vi "MinDisplac(StartP)1.vi"(4 "error IN":errorcluster, 7 "[IN] (X,Y,dX,dY) NN":dbl[][](array[numeric])) -> (0 "error OUT":errorcluster, 3 "[OUT] (X,Y,dX,dY) NN":dbl[][](array[numeric]))   [LabVIEW 2013]
doc: "If origins of displacement have the same coordinates, this subVI saves only minimal"
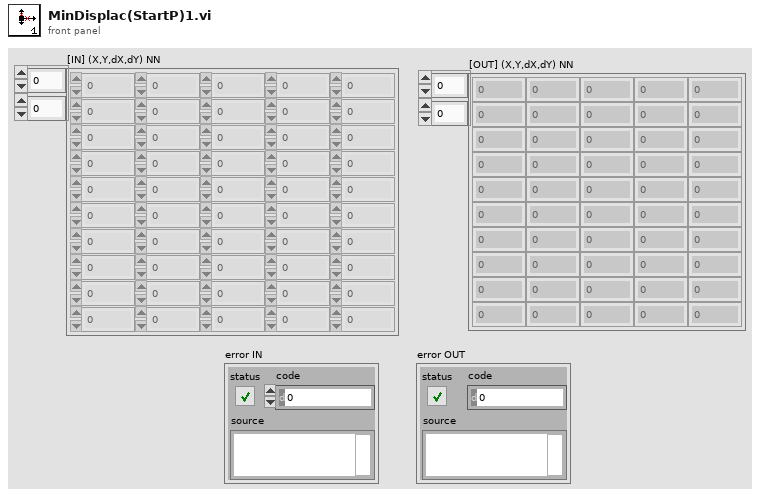
[diagram p1: front panel]
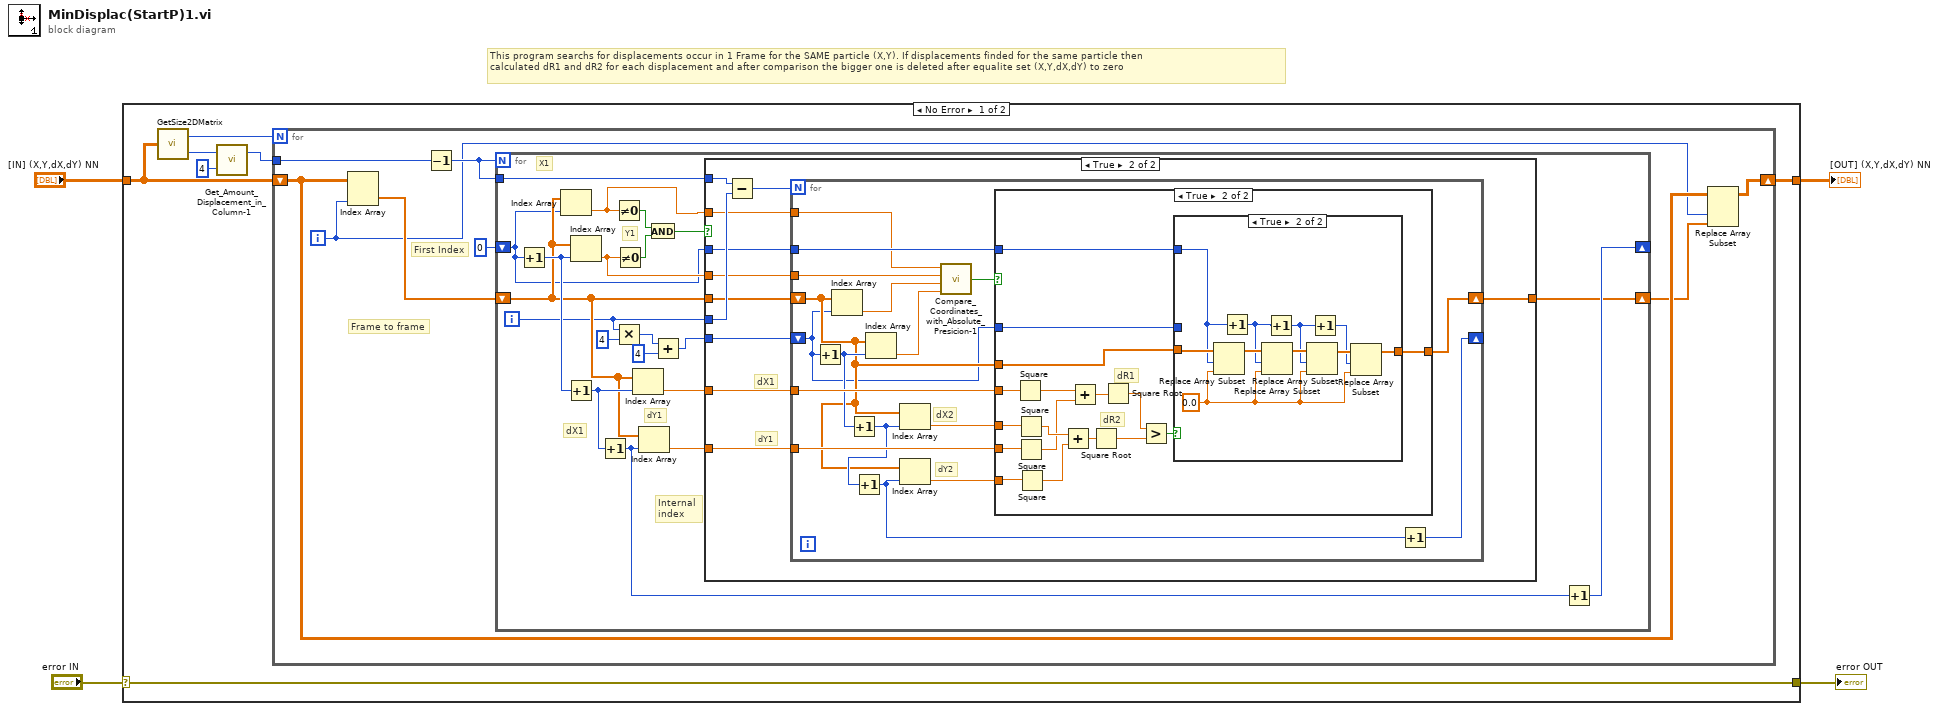
[diagram p0: block diagram]
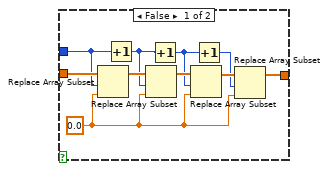
[diagram p4: hidden frame]
diagram:
  # "This program searchs for displacements occur in 1 Frame for the SAME particle (X,Y). If displacements finded for the same particle then \ncalculated dR1 and dR2 for each displacement and after comparison the bigger one is deleted after equalite set (X,Y,dX,dY) to zero"
  n1 = case shown="No Error" "error IN" {
    selector: "error IN" -> [w8 w108]
    tunnel: [w11 w107] -> w4
    tunnel: "[IN] (X,Y,dX,dY) NN" -> [w10 w107]
    tunnel: [w8 w108] -> w1
    frame No Error {
      n2 = call "GetSize2DMatrix.vi"("Array IN (2D)"=w10) -> ("# Cols"=w9:i32, "# Rows"=w7:i32)
      n3 = call "Get_Amount_Displacement_in_Column-1.vi"("multiplier"=4, "# Rows"=w7) -> ("Displ amount"=w5:i32)  [unwired: 1 out]
      n4 = for {
        N: w9 -> [_]
        shift-right: [w13] -> w11
        shift-left: w10 -> [w16]
        tunnel: w5 -> [w12]
        i -> [w15]
        # "First Index"
        # "Frame to frame"
        n5 = Index Array(array=w16, index (col)=w15) -> (element=w19:dbl[])  [unwired: 1 in]
        n6 = Decrement(x=w12) -> (x-1=w17:i32)
        n7 = for {
          N: w17 -> [_]
          shift-right: [w20] -> w14
          shift-left: w19 -> [w31]
          shift-right: [w29] -> _
          shift-left: 0 -> [w21]
          tunnel: w17 -> [w36]
          i -> [w26]
          # "dX1"
          # "dY1"
          # "Internal \nindex"
          # "Y1"
          # "X1"
          n8 = Increment(x=w21) -> (x+1=w33:i32)
          n9 = Index Array(array=w31, index=w21) -> (element=w35:dbl)
          n10 = Increment(x=w33) -> (x+1=w32:i32)
          n11 = Index Array(array=w31, index=w33) -> (element=w34:dbl)
          n12 = Increment(x=w32) -> (x+1=w30:i32)
          n13 = Not Equal To 0?(x=w35) -> (x != 0?=w39:bool)
          n14 = Multiply(x=w26, y=4) -> (x*y=w24:i32)
          n15 = Not Equal To 0?(x=w34) -> (x != 0?=w38:bool)
          n16 = Index Array(array=w31, index=w32) -> (element=w28:dbl)
          n17 = Index Array(array=w31, index=w30) -> (element=w27:dbl)
          n18 = And(x=w39, y=w38) -> (x .and. y?=w37:bool)
          n19 = Add(x=w24, y=4) -> (x+y=w23:i32)
          n20 = case shown="True" w37 {
            tunnel: w36 -> [_ w51]
            tunnel: w26 -> [_ w50]
            tunnel: w35 -> [_ w47]
            tunnel: w34 -> [_ w46]
            tunnel: w31 -> [w40 w48]
            tunnel: [w40 w45] -> w20
            tunnel: w28 -> [_ w44]
            tunnel: w27 -> [_ w43]
            tunnel: w23 -> [_ w42]
            tunnel: w21 -> [_ w41]
            frame False {
            }
            frame True {
              # "dX1"
              # "dY1"
              n21 = Subtract(x=w51, y=w50) -> (x-y=w49:i32)
              n22 = for {
                N: w49 -> [_]
                shift-right: [w58] -> w45
                shift-left: w48 -> [w60]
                tunnel: w47 -> [w54]
                tunnel: w46 -> [w55]
                shift-right: [w61] -> _
                shift-left: w42 -> [w57]
                tunnel: w44 -> [w68]
                tunnel: w43 -> [w67]
                tunnel: w41 -> [w59]
                # "dY2"
                # "dX2"
                n23 = Increment(x=w57) -> (x+1=w66:i32)
                n24 = Index Array(array=w60, index=w57) -> (element=w53:dbl)
                n25 = Increment(x=w66) -> (x+1=w65:i32)
                n26 = Increment(x=w65) -> (x+1=w62:i32)
                n27 = Index Array(array=w60, index=w66) -> (element=w52:dbl)
                n28 = Index Array(array=w60, index=w65) -> (element=w63:dbl)
                n29 = Index Array(array=w60, index=w62) -> (element=w64:dbl)
                n30 = call "Compare_Coordinates_with_Absolute_Presicion-1.vi"("X 1"=w54, "Y 1"=w55, "X 2"=w53, "Y 2"=w52) -> ("[OUT] Same coordinates?"=w56:bool)  [unwired: 1 in]
                n31 = case shown="True" w56 {
                  tunnel: w68 -> [_ w86]
                  tunnel: w67 -> [_ w84]
                  tunnel: w64 -> [_ w83]
                  tunnel: w63 -> [_ w85]
                  tunnel: w60 -> [w69 w76]
                  tunnel: w59 -> [_ w75]
                  tunnel: [w69 w74] -> w58
                  tunnel: w57 -> [_ w73]
                  frame False {
                  }
                  frame True {
                    # "dR2"
                    # "dR1"
                    n32 = Square(x=w86) -> (x^2=w81:dbl)
                    n33 = Square(x=w85) -> (x^2=w72:dbl)
                    n34 = Square(x=w84) -> (x^2=w70:dbl)
                    n35 = Square(x=w83) -> (x^2=w71:dbl)
                    n36 = Add(x=w72, y=w71) -> (x+y=w82:dbl)
                    n37 = Add(x=w81, y=w70) -> (x+y=w80:dbl)
                    n38 = Square Root(x=w82) -> (sqrt(x)=w78:dbl)
                    n39 = Square Root(x=w80) -> (sqrt(x)=w79:dbl)
                    n40 = Greater?(x=w79, y=w78) -> (0:w77:bool)
                    n41 = case shown="True" w77 {
                      tunnel: w76 -> [w89 w106]
                      tunnel: w75 -> [_ w104]
                      tunnel: [w87 w97] -> w74
                      tunnel: w73 -> [w88 _]
                      frame False {
                        w93 = 0.0 ("new element/subarray")
                        n42 = Replace Array Subset(array=w89, new element=w93, index=w88) -> (w96:dbl[])
                        n43 = Increment(x=w88) -> (x+1=w92:i32)
                        n44 = Replace Array Subset(array=w96, new element=w93, index=w92) -> (w95:dbl[])
                        n45 = Increment(x=w92) -> (x+1=w91:i32)
                        n46 = Replace Array Subset(array=w95, new element=w93, index=w91) -> (w94:dbl[])
                        n47 = Increment(x=w91) -> (x+1=w90:i32)
                        n48 = Replace Array Subset(array=w94, new element=w93, index=w90) -> (w87:dbl[])
                      }
                      frame True {
                        w101 = 0.0 ("new element/subarray")
                        n49 = Replace Array Subset(array=w106, new element=w101, index=w104) -> (w105:dbl[])
                        n50 = Increment(x=w104) -> (x+1=w100:i32)
                        n51 = Replace Array Subset(array=w105, new element=w101, index=w100) -> (w103:dbl[])
                        n52 = Increment(x=w100) -> (x+1=w99:i32)
                        n53 = Replace Array Subset(array=w103, new element=w101, index=w99) -> (w102:dbl[])
                        n54 = Increment(x=w99) -> (x+1=w98:i32)
                        n55 = Replace Array Subset(array=w102, new element=w101, index=w98) -> (w97:dbl[])
                      }
                    }
                  }
                }
                n56 = Increment(x=w62) -> (x+1=w61:i32)
              }
            }
          }
          n57 = Increment(x=w30) -> (x+1=w29:i32)
        }
        n58 = Replace Array Subset(array=w16, new element=w14, index (col)=w15) -> (w13:dbl[][])  [unwired: 1 in]
      }
    }
    frame Error {
    }
  }
  "error OUT" <- w1
  "[OUT] (X,Y,dX,dY) NN" <- w4
